vi "varXNode_BuildMenu3.vi"(8 "Click Type":T1, 9 "Point":T2, 10 "XRef":refnum<vi>, 11 "State In":T10) -> (1 "Show Standard Items? (Popup click only)":bool=TRUE, 2 "Menu Specification":T4)   [LabVIEW 2020, in "varXNode.xnode"]
uses:
  <vilib>/variable/varXNode.llb/varXNode.xnode
  <vilib>/variable/varXNode.llb/varXNode.ctl
  <vilib>/variable/Type Descriptor.ctl
  <vilib>/XNodeSupport/XNodeMenuSpecs3.ctl
  <vilib>/XNodeSupport/XNodeMenuSpec3.ctl
  <vilib>/XNodeSupport/XNodeString.ctl
  <vilib>/XNodeSupport/XNodeBool.ctl
  <vilib>/XNodeSupport/XNodeStandardHelpInfo.ctl
  <vilib>/XNodeSupport/XNodePath.ctl
  <vilib>/XNodeSupport/XNodePoint.ctl
  <vilib>/XNodeSupport/XNodeInt.ctl
  <vilib>/XNodeSupport/XNodeClickTypes.ctl
  <vilib>/variable/NI_Variable.lvlib
  <vilib>/XNodeSupport/NI_XNodeSupport.lvlib
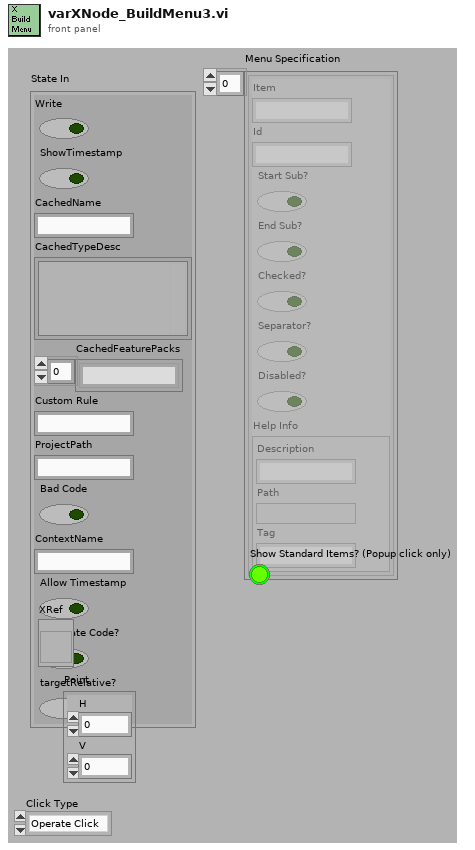
[diagram p1: front panel]
types:
  T1 = typedef "NI_XNodeSupport.lvlib/XNodeClickTypes.ctl" = enum32{"Operate Click", "Popup Click"}
  T2 = typedef "NI_XNodeSupport.lvlib/XNodePoint.ctl" = cluster{"H":T3, "V":T3}
  T3 = typedef "NI_XNodeSupport.lvlib/XNodeInt.ctl" = i32
  T4 = typedef "NI_XNodeSupport.lvlib/XNodeMenuSpecs3.ctl" = T5[]
  T5 = typedef "NI_XNodeSupport.lvlib/XNodeMenuSpec3.ctl" = cluster{"Item":T6, "Id":T6, "Start Sub?":T7, "End Sub?":T7, "Checked?":T7, "Separator?":T7, "Disabled?":T7, "Help Info":T8}
  T6 = typedef "NI_XNodeSupport.lvlib/XNodeString.ctl" = string
  T7 = typedef "NI_XNodeSupport.lvlib/XNodeBool.ctl" = bool
  T8 = typedef "NI_XNodeSupport.lvlib/XNodeStandardHelpInfo.ctl" = cluster{"Description":T6, "Path":T9, "Tag":T6}
  T9 = typedef "NI_XNodeSupport.lvlib/XNodePath.ctl" = path
  T10 = typedef "varXNode.xnode/varXNode.ctl" = cluster{"Write":bool, "ShowTimestamp":bool, "CachedName":string, "CachedTypeDesc":T11, "CachedFeaturePacks":string[], "Custom Rule":string, "ProjectPath":string, "Bad Code":bool, "ContextName":string, "Allow Timestamp":bool, "Generate Code?":bool, "targetRelative?":bool}
  T11 = typedef "NI_Variable.lvlib/Type Descriptor.ctl" = cluster{"Variant":variant}
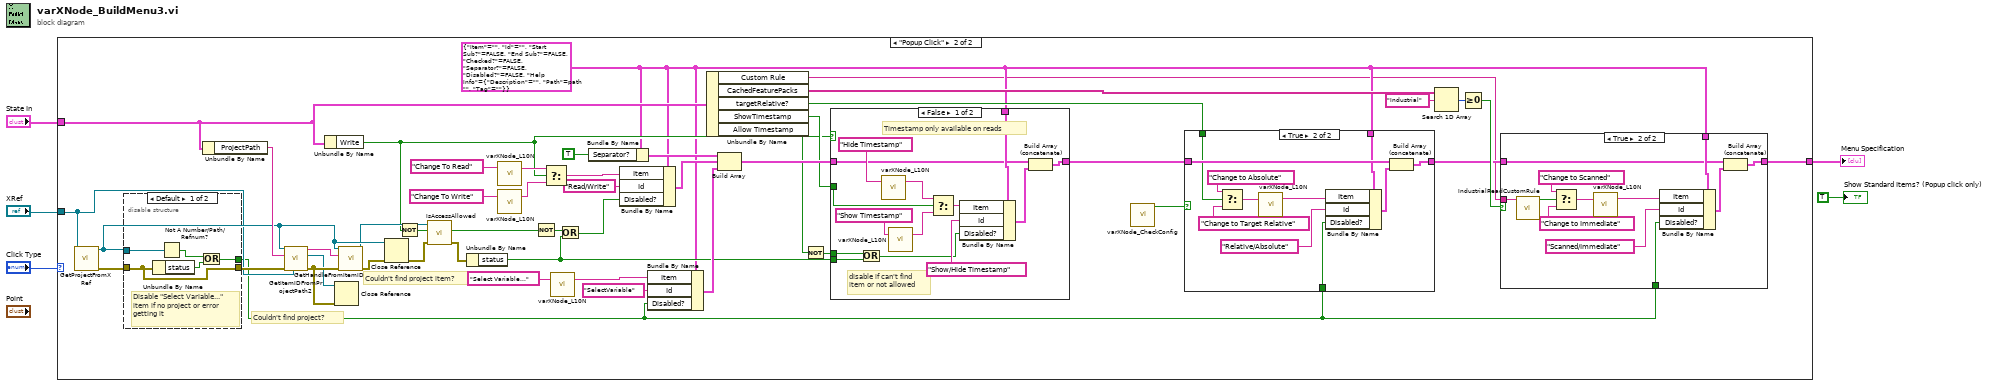
[diagram p0: block diagram]
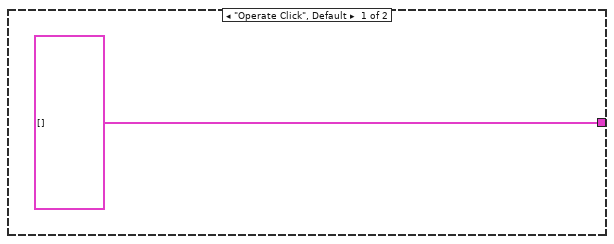
[diagram p2: hidden frame]
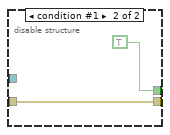
[diagram p6: hidden frame]
diagram:
  n1 = case shown="\"Popup Click\"" "Click Type" {
    tunnel: "XRef" -> [_ w16]
    tunnel: [T5[] [] w10] -> w4
    tunnel: "State In" -> [_ w30]
    frame "Operate Click", Default {
    }
    frame "Popup Click" {
      w9 = T5 {"Item"="", "Id"="", "Start Sub?"=FALSE, "End Sub?"=FALSE, "Checked?"=FALSE, "Separator?"=FALSE, "Disabled?"=FALSE, "Help Info"={"Description"="", "Path"=path "", "Tag"=""}} ("Cluster")
      # "Couldn't find project?"
      # "Couldn't find project item?"
      n2 = call <vilib>:"GetProjectFromXRef.vi"("XRef"=w16) -> ("error out"=w54:errorcluster, "Project"=w48:refnum<vi>)  [unwired: 9 in]
      n3 = disable-structure shown="Default" {
        disable-tunnel: [w99 TRUE ("empty?")] -> w8
        disable-tunnel: w48 -> [w96 _]
        disable-tunnel: w54 -> [w95 w100]
        disable-tunnel: [w95 w100] -> w47
        frame condition #0 (active) {
          # "Disable \"Select Variable...\"\nitem if no project or error\ngetting it"
          n4 = Unbundle By Name(w95) -> ("status"=w97:bool)
          n5 = Not A Number/Path/Refnum?(number/path/refnum=w96) -> (NaN/Path/Refnum?=w98:bool)
          n6 = Or(x=w98, y=w97) -> (x .or. y?=w99:bool)
        }
        frame condition #1 {
        }
      }
      n7 = Unbundle By Name(w30) -> ("ProjectPath"=w53:string)
      n8 = call <vilib>:"GetItemIDFromProjectPath2.vi"("XRef"=w16, "error in"=w47, "ProjectPath"=w53, "Project"=w48) -> ("error out"=w51:errorcluster, "ProjectItem"=w50:refnum<vi>, "Item ID"=w52:string)  [unwired: 5 in]
      n9 = Unbundle By Name(w30) -> ("Write"=w27:bool)
      n10 = Close Reference(reference=w50, error in (no error)=w51) -> ()  [unwired: 1 out]
      n11 = call <vilib>:"GetHandleFromItemID.vi"("error in"=w51, "ItemID"=w52, "Project"=w48) -> ("error out"=w49:errorcluster, "VarHandle"=w28:refnum<k1>)  [unwired: 7 in]
      n12 = Close Reference(reference=w48, error in (no error)=w49) -> (error out=w21:errorcluster)
      n13 = Not(x=w27) -> (.not. x?=w22:bool)
      n14 = call <vilib>:"IsAccessAllowed.vi"("error in (no error)"=w21, "Write?"=w22, "VarHandle in"=w28) -> ("error out"=w20:errorcluster, "Allowed?"=w26:bool)  [unwired: 6 in, 1 out]
      n15 = Unbundle By Name(w20) -> ("status"=w24:bool)
      n16 = call <vilib>:"varXNode_L10N.vi"("String In"="Change To Read" ("item")) -> ("String Out"=w45:string)  [unwired: 2 in]
      n17 = call <vilib>:"varXNode_L10N.vi"("String In"="Change To Write" ("item")) -> ("String Out"=w43:string)  [unwired: 2 in]
      n18 = Not(x=w26) -> (.not. x?=w25:bool)
      n19 = Select(t=w45, s=w27, f=w43) -> (s? t:f=w42:string)
      n20 = call <vilib>:"varXNode_L10N.vi"("String In"="Select Variable..." ("Item")) -> ("String Out"=w39:string)  [unwired: 2 in]
      n21 = Or(x=w25, y=w24) -> (x .or. y?=w23:bool)
      n22 = Bundle By Name(cluster=w9, "Separator?"=TRUE) -> (w36:T5)
      n23 = Bundle By Name(cluster=w9, "Item"=w42, "Id"="Read/Write", "Disabled?"=w23) -> (w35:T5)
      n24 = Bundle By Name(cluster=w9, "Item"=w39, "Id"="SelectVariable", "Disabled?"=w8) -> (w34:T5)
      n25 = Unbundle By Name(w30) -> ("Custom Rule"=w7:string, "CachedFeaturePacks"=w15:string[], "targetRelative?"=w18:bool, "ShowTimestamp"=w31:bool, "Allow Timestamp"=w32:bool)
      n26 = Build Array(w36, w35, w34) -> (w33:T5[])
      n27 = Not(x=w32) -> (.not. x?=w29:bool)
      n28 = case shown="False" w27 {
        tunnel: w33 -> [w82 w94]
        tunnel: w9 -> [w87 _]
        tunnel: w24 -> [w86 _]
        tunnel: w29 -> [w84 _]
        tunnel: w31 -> [w83 _]
        tunnel: [w80 w94] -> w19
        frame False {
          # "disable if can't find\nitem or not allowed"
          # "Timestamp only available on reads"
          n29 = Or(x=w84, y=w86) -> (x .or. y?=w85:bool)
          n30 = call <vilib>:"varXNode_L10N.vi"("String In"="Hide Timestamp" ("Item")) -> ("String Out"=w91:string)  [unwired: 2 in]
          n31 = call <vilib>:"varXNode_L10N.vi"("String In"="Show Timestamp" ("Item")) -> ("String Out"=w90:string)  [unwired: 2 in]
          n32 = Select(t=w91, s=w83, f=w90) -> (s? t:f=w89:string)
          n33 = Bundle By Name(cluster=w87, "Item"=w89, "Id"="Show/Hide Timestamp", "Disabled?"=w85) -> (w81:T5)
          n34 = Build Array (concatenate)(w82, w81) -> (w80:T5[])
        }
        frame True {
        }
      }
      n35 = call <vilib>:"varXNode_CheckConfig.vi"() -> ("Enable Relative Nodes?"=w17:bool)  [unwired: 11 in]
      n36 = case shown="True" w17 {
        tunnel: w19 -> [w68 w79]
        tunnel: w18 -> [_ w77]
        tunnel: w9 -> [_ w74]
        tunnel: w8 -> [_ w73]
        tunnel: [w68 w70] -> w11
        frame False {
        }
        frame True {
          n37 = Select(t="Change to Absolute", s=w77, f="Change to Target Relative") -> (s? t:f=w78:string)
          n38 = call <vilib>:"varXNode_L10N.vi"("String In"=w78) -> ("String Out"=w72:string)  [unwired: 2 in]
          n39 = Bundle By Name(cluster=w74, "Item"=w72, "Id"=T6 "Relative/Absolute", "Disabled?"=w73) -> (w69:T5)
          n40 = Build Array (concatenate)(w79, w69) -> (w70:T5[])
        }
      }
      n41 = Search 1D Array(1D array=w15, element="Industrial") -> (index of element=w13:i32)  [unwired: 1 in]
      n42 = Greater Or Equal To 0?(x=w13) -> (x >= 0?=w12:bool)
      n43 = case shown="True" w12 {
        tunnel: w11 -> [w55 w59]
        tunnel: [w55 w58] -> w10
        tunnel: w9 -> [_ w61]
        tunnel: w8 -> [_ w60]
        tunnel: w7 -> [_ w57]
        frame False {
        }
        frame True {
          n44 = call <vilib>:"IndustrialReadCustomRule.vi"("Custom Rule"=w57) -> ("IsImmediate"=w56:bool)  [unwired: 10 in]
          n45 = Select(t="Change to Scanned", s=w56, f="Change to Immediate") -> (s? t:f=w62:string)
          n46 = call <vilib>:"varXNode_L10N.vi"("String In"=w62) -> ("String Out"=w65:string)  [unwired: 2 in]
          n47 = Bundle By Name(cluster=w61, "Item"=w65, "Id"=T6 "Scanned/Immediate", "Disabled?"=w60) -> (w67:T5)
          n48 = Build Array (concatenate)(w59, w67) -> (w58:T5[])
        }
      }
    }
  }
  "Menu Specification" <- w4
  "Show Standard Items? (Popup click only)" <- TRUE ("Show Standard Items? (Popup click only)")
